vi "Conrol-s-de-activate.vi"   [LabVIEW 2015]
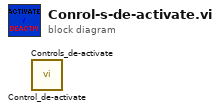
[diagram p0: block diagram]
diagram:
  n1 = call "Control_de-activate.vi"() -> ()  [unwired: 2 in]
  n2 = call "Controls_de-activate.vi"() -> ()  [unwired: 2 in]
